vi "Set Intensity Scales (Start and End).vi"(7 "IntensityGraph in":refnum<vi>, 8 "error in (no error)":errorcluster, 9 "y start & end":cluster{"y start":dbl, "y end":dbl}, 10 "x start & end":cluster{"x start":dbl, "x end":dbl}, 11 "Intensity Data":dbl[][](array[numeric])) -> (0 "error out":errorcluster)   [LabVIEW 2016, in "graph_utilities.lvlib"]
uses:
  <vilib>/Utility/miscctls.llb/LVOffsetAndMultiplierTypeDef.ctl
  graph_utilities.lvlib
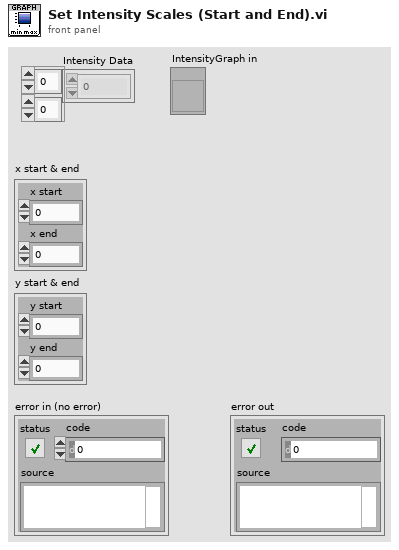
[diagram p1: front panel]
types:
  T1 = typedef "LVOffsetAndMultiplierTypeDef.ctl" = cluster{"Offset":dbl, "Multiplier":dbl}
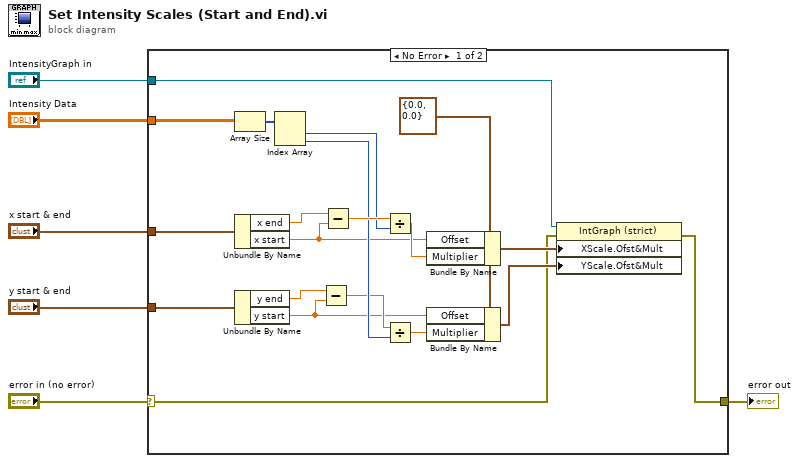
[diagram p0: block diagram]
diagram:
  n1 = case shown="No Error" "error in (no error)" {
    selector: "error in (no error)" -> [w12 w27]
    tunnel: "Intensity Data" -> [w22 _]
    tunnel: "IntensityGraph in" -> [w21 _]
    tunnel: "x start & end" -> [w20 _]
    tunnel: "y start & end" -> [w18 _]
    tunnel: [w13 w27] -> w2
    frame No Error {
      w14 = T1 {"Offset"=0.0, "Multiplier"=0.0} ("X Scale.Offset and Multiplier")
      n2 = Array Size(array=w22) -> (size(s)=w23:i32[])
      n3 = Unbundle By Name(w20) -> ("x end"=w19:dbl, "x start"=w9:dbl)
      n4 = Unbundle By Name(w18) -> ("y end"=w17:dbl, "y start"=w7:dbl)
      n5 = Index Array(array=w23) -> (element #1=w10:i32, element #2=w16:i32)  [unwired: 2 in]
      n6 = Subtract(x=w17, y=w7) -> (x-y=w8:dbl)
      n7 = Subtract(x=w19, y=w9) -> (x-y=w24:dbl)
      n8 = Divide(x=w24, y=w10) -> (x/y=w11:dbl)
      n9 = Divide(x=w8, y=w16) -> (x/y=w25:dbl)
      n10 = Bundle By Name(cluster=w14, "Offset"=w9, "Multiplier"=w11) -> (w26:T1)
      n11 = Bundle By Name(cluster=w14, "Offset"=w7, "Multiplier"=w25) -> (w15:T1)
      n12 = property on="Property Node" class="IntGraph (strict)"(reference=w21, error in=w12, "XScale.Ofst&Mult"=w26, "YScale.Ofst&Mult"=w15) -> (error out=w13:errorcluster)  [unwired: 1 out]
    }
    frame Error {
    }
  }
  "error out" <- w2
